vi "6.3.25 xfb.vi"() -> ()   [LabVIEW 2020]
uses:
  5fafc9fc-07f3-418d-bf4a-bd53c0c0d1ca.vi
  81c18395-6a0c-4167-8ea2-1033434bdb76.vi
  <vilib>/Comparison/Less/Less Functor/Less Functor.lvclass
panel:
  out "decimal integer string":string
  out "o/p 2":string
  in  "Numeric":dbl
  out "sum 2":dbl
  out "sorted array":dbl[](array[numeric])
  out "Array 2":dbl[](array[numeric])
  out "o/p":string
  out "sum":dbl
  in  "i/p":dbl
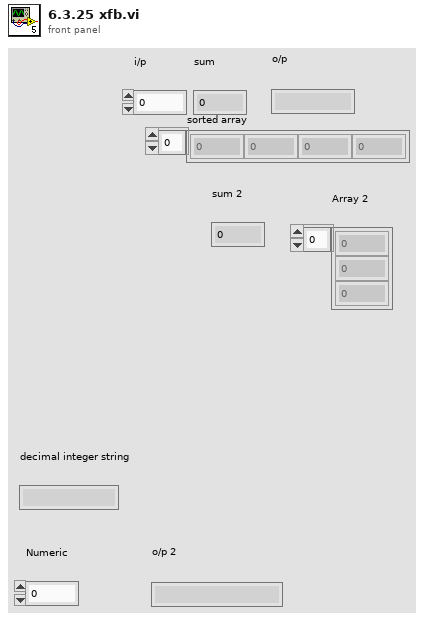
[diagram p1: front panel]
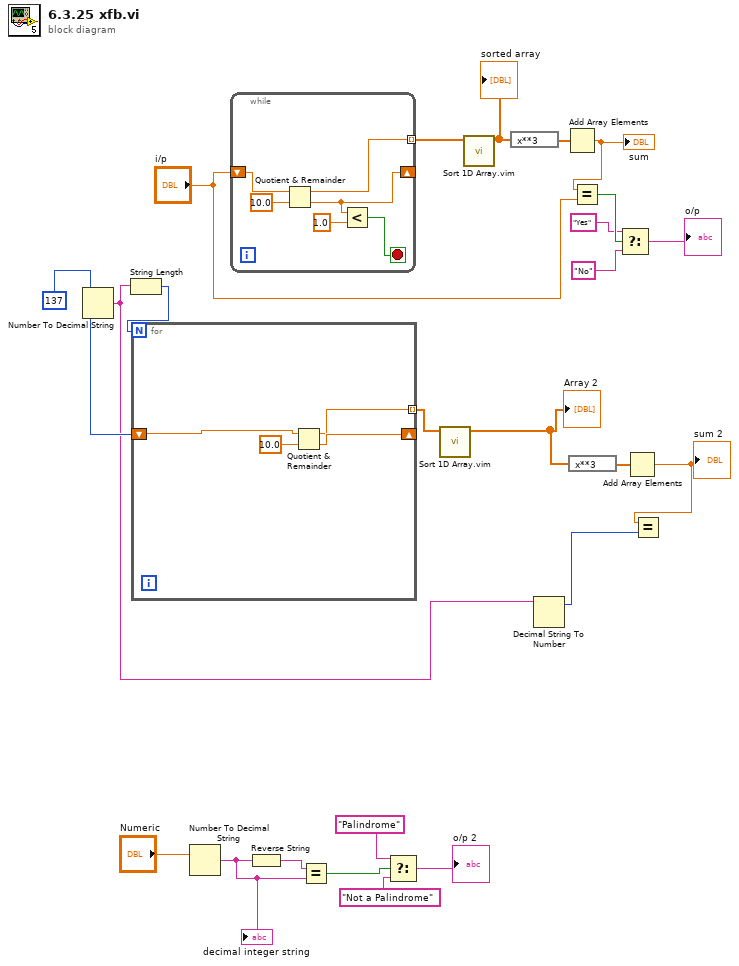
[diagram p0: block diagram]
diagram:
  w14 = 137
  n1 = Number To Decimal String(number=w14) -> (decimal integer string=w9:string)  [unwired: 1 in]
  n2 = String Length(string=w9) -> (length=w15:i32)
  n3 = for {
    N: w15 -> [_]
    shift-right: [w26] -> _
    shift-left: w14 -> [w27]
    tunnel: [w25] -> w13 mode=indexing
    n4 = Quotient & Remainder(x=w27, y=10.0) -> (x-y*floor(x/y)=w25:dbl, floor(x/y)=w26:dbl)
  }
  n5 = Number To Decimal String(number="Numeric") -> (decimal integer string=w6:string)  [unwired: 1 in]
  "decimal integer string" <- w6
  n6 = while {
    shift-right: [w30] -> _
    shift-left: "i/p" -> [w34]
    tunnel: [w32] -> w24 mode=indexing
    stop <- w29 stop-if-true
    n7 = Quotient & Remainder(x=w34, y=10.0) -> (x-y*floor(x/y)=w32:dbl, floor(x/y)=w30:dbl)
    n8 = Less?(x=w30, y=1.0) -> (x < y?=w29:bool)
  }
  n9 = Reverse String(1:w6) -> (0:w7:string)
  n10 = Equal?(x=w7, y=w6) -> (x = y?=w1:bool)
  n11 = Select(t="Palindrome", s=w1, f="Not a Palindrome") -> (s? t:f=→"o/p 2":string)
  n12 = call "Sort 1D Array.vim"("unsorted array"=w13) -> ("sorted array"=w11:dbl[])  [unwired: 10 in]
  "Array 2" <- w11
  n13 = call "Sort 1D Array.vim"("unsorted array"=w24) -> ("sorted array"=w23:dbl[])  [unwired: 10 in]
  "sorted array" <- w23
  n14 = expression code="x**3"(w23) -> (w22:dbl[])
  n15 = Decimal String To Number(string=w9) -> (offset past number=w8:i32)  [unwired: 2 in, 1 out]
  n16 = Add Array Elements(numeric array=w22) -> (sum=w21:dbl)
  "sum" <- w21
  n17 = expression code="x**3"(w11) -> (w12:dbl[])
  n18 = Equal?(x=w21, y="i/p") -> (x = y?=w18:bool)
  n19 = Select(t="Yes", s=w18, f="No") -> (s? t:f=→"o/p":string)
  n20 = Add Array Elements(numeric array=w12) -> (sum=w10:dbl)
  "sum 2" <- w10
  n21 = Equal?(x=w10, y=w8) -> ()  [unwired: 1 out]
